vi "击打按钮.vi"(2 "Get_Di_通道号":u8=1 min=1 max=8) -> (0 "返回值（点亮为返回T）":bool)   [LabVIEW 2010]
panel:
  in  "部位 8":bool
  in  "部位 7":bool
  in  "部位 6":bool
  in  "部位 5":bool
  in  "部位 4":bool
  in  "部位 3":bool
  in  "部位 2":bool
  in  "部位1":bool
  # "*按下时值为真"
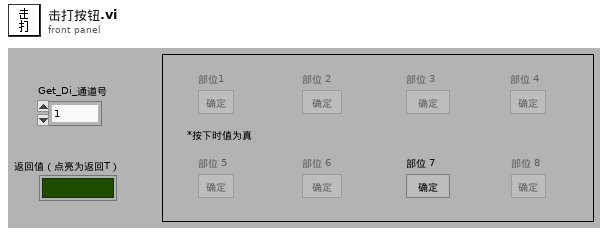
[diagram p1: front panel]
types:
  T1 = enum8{"Enabled", "Disabled", "Disabled and Grayed Out"}
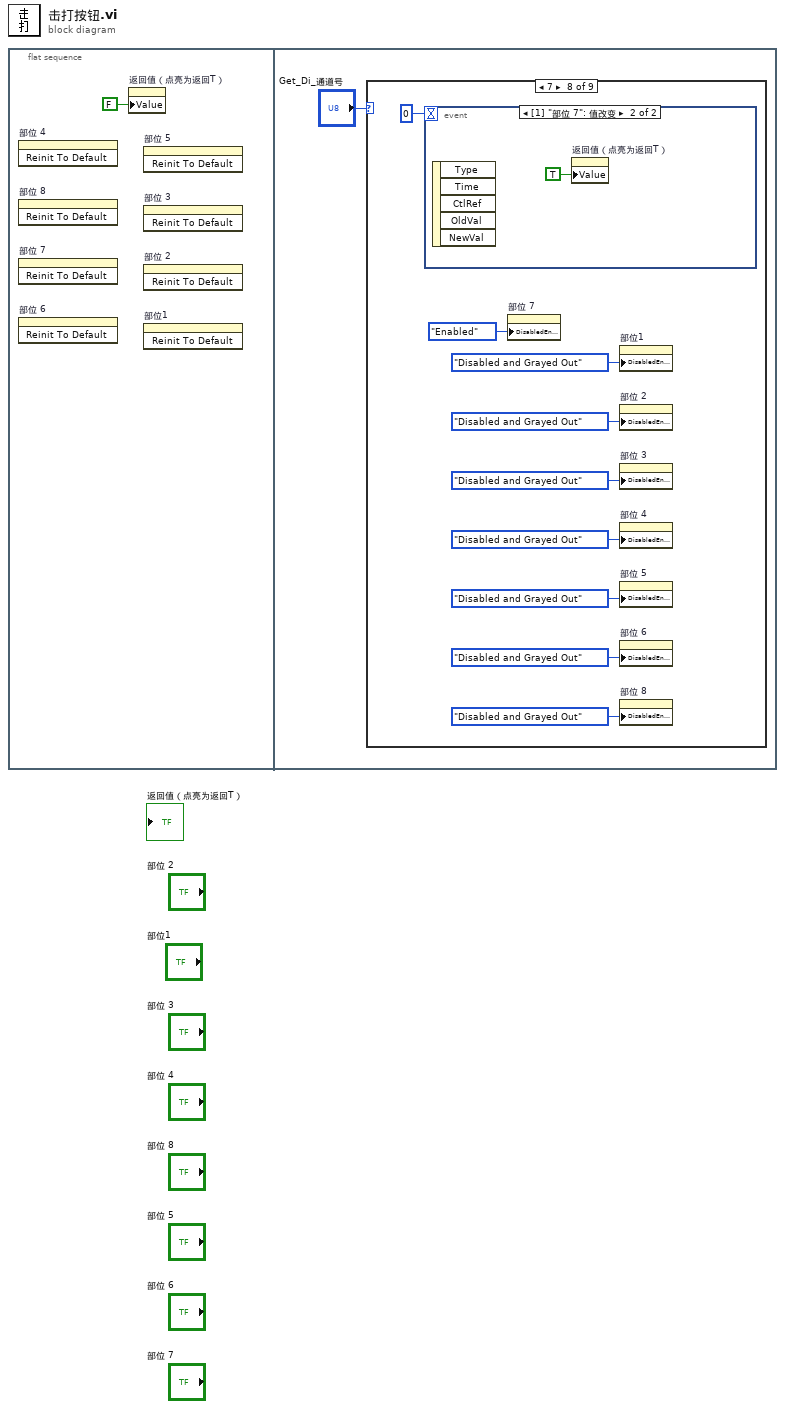
[diagram p0: block diagram]
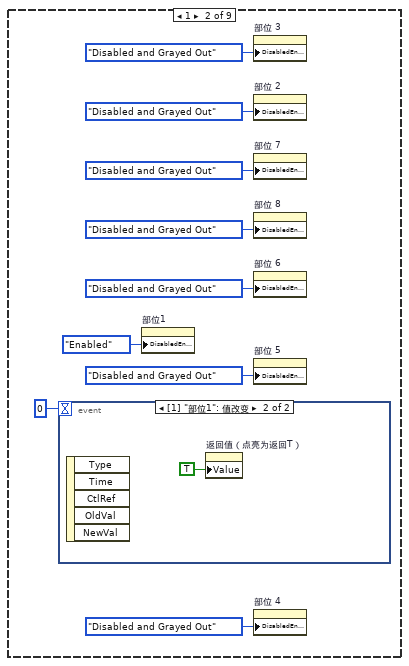
[diagram p3: hidden frame]
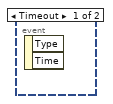
[diagram p4: hidden frame]
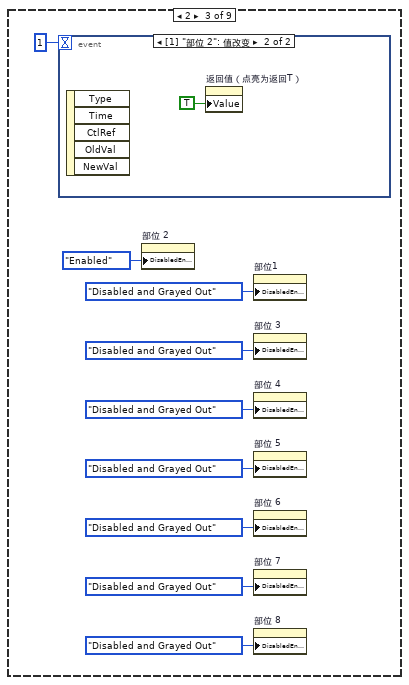
[diagram p5: hidden frame]
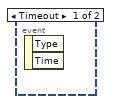
[diagram p6: hidden frame]
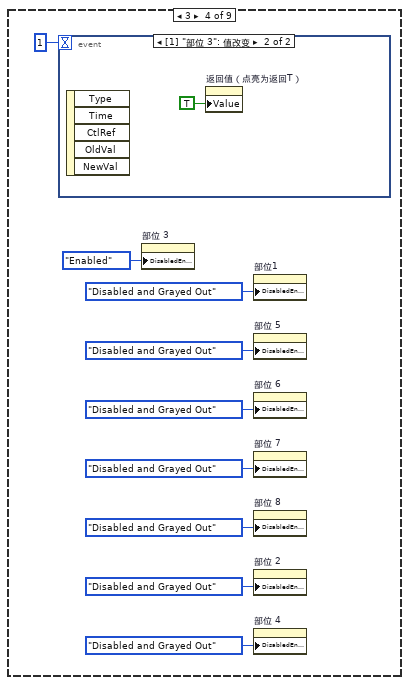
[diagram p7: hidden frame]
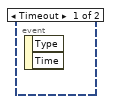
[diagram p8: hidden frame]
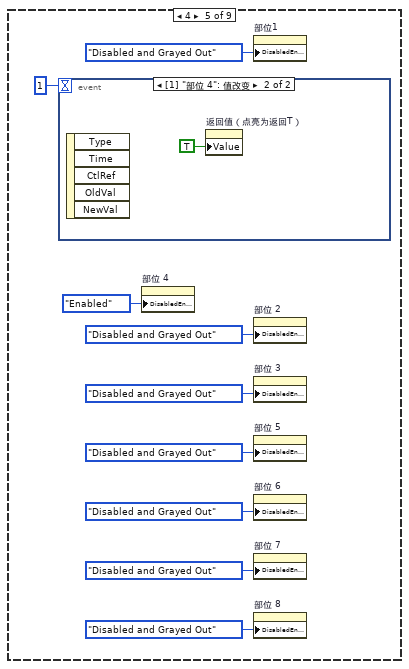
[diagram p9: hidden frame]
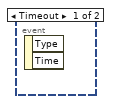
[diagram p10: hidden frame]
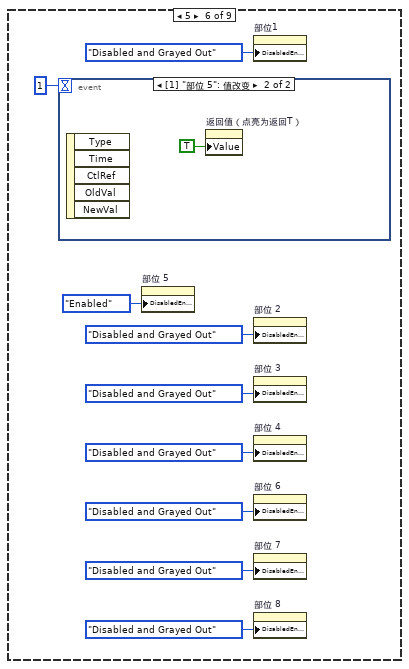
[diagram p11: hidden frame]
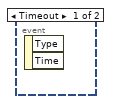
[diagram p12: hidden frame]
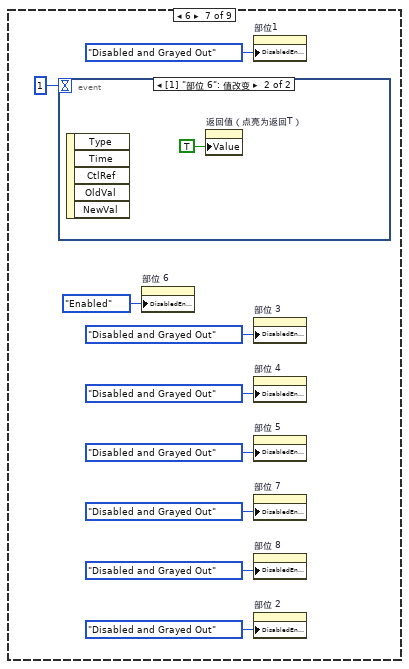
[diagram p13: hidden frame]
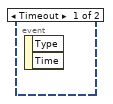
[diagram p14: hidden frame]
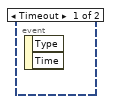
[diagram p15: hidden frame]
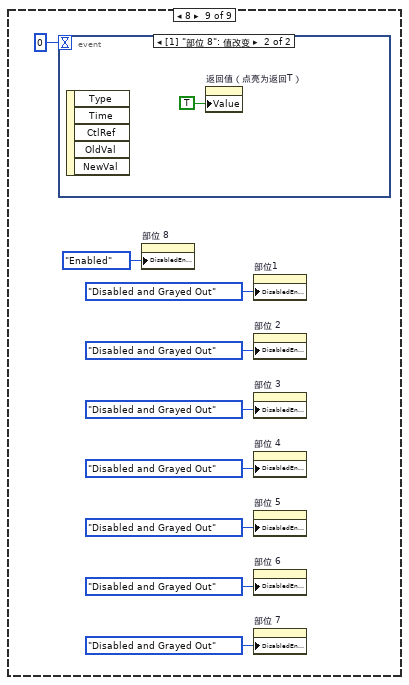
[diagram p16: hidden frame]
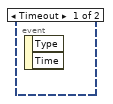
[diagram p17: hidden frame]
diagram:
  n1 = flat-sequence {
    frame #0 {
      n2 = invoke on="部位 4" class="Bool" method="Reinit To Default"() -> ()  [unwired: 3 in, 3 out]
      n3 = invoke on="部位 8" class="Bool" method="Reinit To Default"() -> ()  [unwired: 3 in, 3 out]
      n4 = invoke on="部位 7" class="Bool" method="Reinit To Default"() -> ()  [unwired: 3 in, 3 out]
      n5 = invoke on="部位 6" class="Bool" method="Reinit To Default"() -> ()  [unwired: 3 in, 3 out]
      n6 = property on="返回值（点亮为返回T）" class="Bool (严格)"("Value"=FALSE ("返回值")) -> ()  [unwired: 2 in, 2 out]
      n7 = invoke on="部位 5" class="Bool" method="Reinit To Default"() -> ()  [unwired: 3 in, 3 out]
      n8 = invoke on="部位 3" class="Bool" method="Reinit To Default"() -> ()  [unwired: 3 in, 3 out]
      n9 = invoke on="部位 2" class="Bool" method="Reinit To Default"() -> ()  [unwired: 3 in, 3 out]
      n10 = invoke on="部位1" class="Bool" method="Reinit To Default"() -> ()  [unwired: 3 in, 3 out]
    }
    frame #1 {
      n11 = case shown="7" "Get_Di_通道号" {
        frame 0, Default {
        }
        frame 1 {
          n12 = event shown="[1] \"部位1\": 值改变" {
            selector: _ -> [_ _]
            dyn-events: _ -> [_ _]
            timeout: 0 -> [_ _]
            event Timeout {
              n13 = event-data() -> ()  [unwired: 1 in, 2 out]
            }
            event "部位1": Value Change {
              n14 = event-data() -> ()  [unwired: 1 in, 5 out]
              n15 = property on="返回值（点亮为返回T）" class="Bool (严格)"("Value"=TRUE ("灯1")) -> ()  [unwired: 2 in, 2 out]
            }
          }
          n16 = property on="部位1" class="Bool"("DisabledEnum"=T1."Enabled" ("禁用")) -> ()  [unwired: 2 in, 2 out]
          n17 = property on="部位 3" class="Bool"("DisabledEnum"=T1."Disabled and Grayed Out" ("禁用")) -> ()  [unwired: 2 in, 2 out]
          n18 = property on="部位 2" class="Bool"("DisabledEnum"=T1."Disabled and Grayed Out" ("禁用")) -> ()  [unwired: 2 in, 2 out]
          n19 = property on="部位 7" class="Bool"("DisabledEnum"=T1."Disabled and Grayed Out" ("禁用")) -> ()  [unwired: 2 in, 2 out]
          n20 = property on="部位 8" class="Bool"("DisabledEnum"=T1."Disabled and Grayed Out" ("禁用")) -> ()  [unwired: 2 in, 2 out]
          n21 = property on="部位 6" class="Bool"("DisabledEnum"=T1."Disabled and Grayed Out" ("禁用")) -> ()  [unwired: 2 in, 2 out]
          n22 = property on="部位 5" class="Bool"("DisabledEnum"=T1."Disabled and Grayed Out" ("禁用")) -> ()  [unwired: 2 in, 2 out]
          n23 = property on="部位 4" class="Bool"("DisabledEnum"=T1."Disabled and Grayed Out" ("禁用")) -> ()  [unwired: 2 in, 2 out]
        }
        frame 2 {
          n24 = event shown="[1] \"部位 2\": 值改变" {
            selector: _ -> [_ _]
            dyn-events: _ -> [_ _]
            timeout: 1 -> [_ _]
            event Timeout {
              n25 = event-data() -> ()  [unwired: 1 in, 2 out]
            }
            event "部位 2": Value Change {
              n26 = event-data() -> ()  [unwired: 1 in, 5 out]
              n27 = property on="返回值（点亮为返回T）" class="Bool (严格)"("Value"=TRUE ("灯2")) -> ()  [unwired: 2 in, 2 out]
            }
          }
          n28 = property on="部位 2" class="Bool"("DisabledEnum"=T1."Enabled" ("禁用")) -> ()  [unwired: 2 in, 2 out]
          n29 = property on="部位1" class="Bool"("DisabledEnum"=T1."Disabled and Grayed Out" ("禁用")) -> ()  [unwired: 2 in, 2 out]
          n30 = property on="部位 3" class="Bool"("DisabledEnum"=T1."Disabled and Grayed Out" ("禁用")) -> ()  [unwired: 2 in, 2 out]
          n31 = property on="部位 4" class="Bool"("DisabledEnum"=T1."Disabled and Grayed Out" ("禁用")) -> ()  [unwired: 2 in, 2 out]
          n32 = property on="部位 5" class="Bool"("DisabledEnum"=T1."Disabled and Grayed Out" ("禁用")) -> ()  [unwired: 2 in, 2 out]
          n33 = property on="部位 6" class="Bool"("DisabledEnum"=T1."Disabled and Grayed Out" ("禁用")) -> ()  [unwired: 2 in, 2 out]
          n34 = property on="部位 7" class="Bool"("DisabledEnum"=T1."Disabled and Grayed Out" ("禁用")) -> ()  [unwired: 2 in, 2 out]
          n35 = property on="部位 8" class="Bool"("DisabledEnum"=T1."Disabled and Grayed Out" ("禁用")) -> ()  [unwired: 2 in, 2 out]
        }
        frame 3 {
          n36 = event shown="[1] \"部位 3\": 值改变" {
            selector: _ -> [_ _]
            dyn-events: _ -> [_ _]
            timeout: 1 -> [_ _]
            event Timeout {
              n37 = event-data() -> ()  [unwired: 1 in, 2 out]
            }
            event "部位 3": Value Change {
              n38 = event-data() -> ()  [unwired: 1 in, 5 out]
              n39 = property on="返回值（点亮为返回T）" class="Bool (严格)"("Value"=TRUE ("灯3")) -> ()  [unwired: 2 in, 2 out]
            }
          }
          n40 = property on="部位 3" class="Bool"("DisabledEnum"=T1."Enabled" ("禁用")) -> ()  [unwired: 2 in, 2 out]
          n41 = property on="部位1" class="Bool"("DisabledEnum"=T1."Disabled and Grayed Out" ("禁用")) -> ()  [unwired: 2 in, 2 out]
          n42 = property on="部位 5" class="Bool"("DisabledEnum"=T1."Disabled and Grayed Out" ("禁用")) -> ()  [unwired: 2 in, 2 out]
          n43 = property on="部位 6" class="Bool"("DisabledEnum"=T1."Disabled and Grayed Out" ("禁用")) -> ()  [unwired: 2 in, 2 out]
          n44 = property on="部位 7" class="Bool"("DisabledEnum"=T1."Disabled and Grayed Out" ("禁用")) -> ()  [unwired: 2 in, 2 out]
          n45 = property on="部位 8" class="Bool"("DisabledEnum"=T1."Disabled and Grayed Out" ("禁用")) -> ()  [unwired: 2 in, 2 out]
          n46 = property on="部位 2" class="Bool"("DisabledEnum"=T1."Disabled and Grayed Out" ("禁用")) -> ()  [unwired: 2 in, 2 out]
          n47 = property on="部位 4" class="Bool"("DisabledEnum"=T1."Disabled and Grayed Out" ("禁用")) -> ()  [unwired: 2 in, 2 out]
        }
        frame 4 {
          n48 = event shown="[1] \"部位 4\": 值改变" {
            selector: _ -> [_ _]
            dyn-events: _ -> [_ _]
            timeout: 1 -> [_ _]
            event Timeout {
              n49 = event-data() -> ()  [unwired: 1 in, 2 out]
            }
            event "部位 4": Value Change {
              n50 = event-data() -> ()  [unwired: 1 in, 5 out]
              n51 = property on="返回值（点亮为返回T）" class="Bool (严格)"("Value"=TRUE ("灯4")) -> ()  [unwired: 2 in, 2 out]
            }
          }
          n52 = property on="部位 4" class="Bool"("DisabledEnum"=T1."Enabled" ("禁用")) -> ()  [unwired: 2 in, 2 out]
          n53 = property on="部位1" class="Bool"("DisabledEnum"=T1."Disabled and Grayed Out" ("禁用")) -> ()  [unwired: 2 in, 2 out]
          n54 = property on="部位 2" class="Bool"("DisabledEnum"=T1."Disabled and Grayed Out" ("禁用")) -> ()  [unwired: 2 in, 2 out]
          n55 = property on="部位 3" class="Bool"("DisabledEnum"=T1."Disabled and Grayed Out" ("禁用")) -> ()  [unwired: 2 in, 2 out]
          n56 = property on="部位 5" class="Bool"("DisabledEnum"=T1."Disabled and Grayed Out" ("禁用")) -> ()  [unwired: 2 in, 2 out]
          n57 = property on="部位 6" class="Bool"("DisabledEnum"=T1."Disabled and Grayed Out" ("禁用")) -> ()  [unwired: 2 in, 2 out]
          n58 = property on="部位 7" class="Bool"("DisabledEnum"=T1."Disabled and Grayed Out" ("禁用")) -> ()  [unwired: 2 in, 2 out]
          n59 = property on="部位 8" class="Bool"("DisabledEnum"=T1."Disabled and Grayed Out" ("禁用")) -> ()  [unwired: 2 in, 2 out]
        }
        frame 5 {
          n60 = event shown="[1] \"部位 5\": 值改变" {
            selector: _ -> [_ _]
            dyn-events: _ -> [_ _]
            timeout: 1 -> [_ _]
            event Timeout {
              n61 = event-data() -> ()  [unwired: 1 in, 2 out]
            }
            event "部位 5": Value Change {
              n62 = event-data() -> ()  [unwired: 1 in, 5 out]
              n63 = property on="返回值（点亮为返回T）" class="Bool (严格)"("Value"=TRUE ("灯5")) -> ()  [unwired: 2 in, 2 out]
            }
          }
          n64 = property on="部位 5" class="Bool"("DisabledEnum"=T1."Enabled" ("禁用")) -> ()  [unwired: 2 in, 2 out]
          n65 = property on="部位1" class="Bool"("DisabledEnum"=T1."Disabled and Grayed Out" ("禁用")) -> ()  [unwired: 2 in, 2 out]
          n66 = property on="部位 2" class="Bool"("DisabledEnum"=T1."Disabled and Grayed Out" ("禁用")) -> ()  [unwired: 2 in, 2 out]
          n67 = property on="部位 3" class="Bool"("DisabledEnum"=T1."Disabled and Grayed Out" ("禁用")) -> ()  [unwired: 2 in, 2 out]
          n68 = property on="部位 4" class="Bool"("DisabledEnum"=T1."Disabled and Grayed Out" ("禁用")) -> ()  [unwired: 2 in, 2 out]
          n69 = property on="部位 6" class="Bool"("DisabledEnum"=T1."Disabled and Grayed Out" ("禁用")) -> ()  [unwired: 2 in, 2 out]
          n70 = property on="部位 7" class="Bool"("DisabledEnum"=T1."Disabled and Grayed Out" ("禁用")) -> ()  [unwired: 2 in, 2 out]
          n71 = property on="部位 8" class="Bool"("DisabledEnum"=T1."Disabled and Grayed Out" ("禁用")) -> ()  [unwired: 2 in, 2 out]
        }
        frame 6 {
          n72 = event shown="[1] \"部位 6\": 值改变" {
            selector: _ -> [_ _]
            dyn-events: _ -> [_ _]
            timeout: 1 -> [_ _]
            event Timeout {
              n73 = event-data() -> ()  [unwired: 1 in, 2 out]
            }
            event "部位 6": Value Change {
              n74 = event-data() -> ()  [unwired: 1 in, 5 out]
              n75 = property on="返回值（点亮为返回T）" class="Bool (严格)"("Value"=TRUE ("灯6")) -> ()  [unwired: 2 in, 2 out]
            }
          }
          n76 = property on="部位 6" class="Bool"("DisabledEnum"=T1."Enabled" ("禁用")) -> ()  [unwired: 2 in, 2 out]
          n77 = property on="部位1" class="Bool"("DisabledEnum"=T1."Disabled and Grayed Out" ("禁用")) -> ()  [unwired: 2 in, 2 out]
          n78 = property on="部位 3" class="Bool"("DisabledEnum"=T1."Disabled and Grayed Out" ("禁用")) -> ()  [unwired: 2 in, 2 out]
          n79 = property on="部位 4" class="Bool"("DisabledEnum"=T1."Disabled and Grayed Out" ("禁用")) -> ()  [unwired: 2 in, 2 out]
          n80 = property on="部位 5" class="Bool"("DisabledEnum"=T1."Disabled and Grayed Out" ("禁用")) -> ()  [unwired: 2 in, 2 out]
          n81 = property on="部位 7" class="Bool"("DisabledEnum"=T1."Disabled and Grayed Out" ("禁用")) -> ()  [unwired: 2 in, 2 out]
          n82 = property on="部位 8" class="Bool"("DisabledEnum"=T1."Disabled and Grayed Out" ("禁用")) -> ()  [unwired: 2 in, 2 out]
          n83 = property on="部位 2" class="Bool"("DisabledEnum"=T1."Disabled and Grayed Out" ("禁用")) -> ()  [unwired: 2 in, 2 out]
        }
        frame 7 {
          n84 = event shown="[1] \"部位 7\": 值改变" {
            selector: _ -> [_ _]
            dyn-events: _ -> [_ _]
            timeout: 0 -> [_ _]
            event Timeout {
              n85 = event-data() -> ()  [unwired: 1 in, 2 out]
            }
            event "部位 7": Value Change {
              n86 = event-data() -> ()  [unwired: 1 in, 5 out]
              n87 = property on="返回值（点亮为返回T）" class="Bool (严格)"("Value"=TRUE ("灯7")) -> ()  [unwired: 2 in, 2 out]
            }
          }
          n88 = property on="部位 7" class="Bool"("DisabledEnum"=T1."Enabled" ("禁用")) -> ()  [unwired: 2 in, 2 out]
          n89 = property on="部位1" class="Bool"("DisabledEnum"=T1."Disabled and Grayed Out" ("禁用")) -> ()  [unwired: 2 in, 2 out]
          n90 = property on="部位 2" class="Bool"("DisabledEnum"=T1."Disabled and Grayed Out" ("禁用")) -> ()  [unwired: 2 in, 2 out]
          n91 = property on="部位 3" class="Bool"("DisabledEnum"=T1."Disabled and Grayed Out" ("禁用")) -> ()  [unwired: 2 in, 2 out]
          n92 = property on="部位 4" class="Bool"("DisabledEnum"=T1."Disabled and Grayed Out" ("禁用")) -> ()  [unwired: 2 in, 2 out]
          n93 = property on="部位 5" class="Bool"("DisabledEnum"=T1."Disabled and Grayed Out" ("禁用")) -> ()  [unwired: 2 in, 2 out]
          n94 = property on="部位 6" class="Bool"("DisabledEnum"=T1."Disabled and Grayed Out" ("禁用")) -> ()  [unwired: 2 in, 2 out]
          n95 = property on="部位 8" class="Bool"("DisabledEnum"=T1."Disabled and Grayed Out" ("禁用")) -> ()  [unwired: 2 in, 2 out]
        }
        frame 8 {
          n96 = event shown="[1] \"部位 8\": 值改变" {
            selector: _ -> [_ _]
            dyn-events: _ -> [_ _]
            timeout: 0 -> [_ _]
            event Timeout {
              n97 = event-data() -> ()  [unwired: 1 in, 2 out]
            }
            event "部位 8": Value Change {
              n98 = event-data() -> ()  [unwired: 1 in, 5 out]
              n99 = property on="返回值（点亮为返回T）" class="Bool (严格)"("Value"=TRUE ("灯8")) -> ()  [unwired: 2 in, 2 out]
            }
          }
          n100 = property on="部位 8" class="Bool"("DisabledEnum"=T1."Enabled" ("禁用")) -> ()  [unwired: 2 in, 2 out]
          n101 = property on="部位1" class="Bool"("DisabledEnum"=T1."Disabled and Grayed Out" ("禁用")) -> ()  [unwired: 2 in, 2 out]
          n102 = property on="部位 2" class="Bool"("DisabledEnum"=T1."Disabled and Grayed Out" ("禁用")) -> ()  [unwired: 2 in, 2 out]
          n103 = property on="部位 3" class="Bool"("DisabledEnum"=T1."Disabled and Grayed Out" ("禁用")) -> ()  [unwired: 2 in, 2 out]
          n104 = property on="部位 4" class="Bool"("DisabledEnum"=T1."Disabled and Grayed Out" ("禁用")) -> ()  [unwired: 2 in, 2 out]
          n105 = property on="部位 5" class="Bool"("DisabledEnum"=T1."Disabled and Grayed Out" ("禁用")) -> ()  [unwired: 2 in, 2 out]
          n106 = property on="部位 6" class="Bool"("DisabledEnum"=T1."Disabled and Grayed Out" ("禁用")) -> ()  [unwired: 2 in, 2 out]
          n107 = property on="部位 7" class="Bool"("DisabledEnum"=T1."Disabled and Grayed Out" ("禁用")) -> ()  [unwired: 2 in, 2 out]
        }
      }
    }
  }
